vi "simArbSignal_rampUp.vi"(8 "error in (no error)":errorcluster, 9 "Reset":bool, 10 "Next Value":bool=TRUE) -> (0 "error out":errorcluster, 2 "Data Valid":bool, 3 "Signal":dynamicdata(graph)=[{"t0"=timestamp(0 s since 1904-01-01), "dt"=0.5, "Y"=array[3614 elements], "attributes"=variant("NI_ChannelName"=variant(string "Signal"))}])   [LabVIEW 2017]
doc: "Simulates a signal that you define.\n--------------------\n\nThis Express VI is configured as follows:\n\nMode: Packet (The whole waveform each run)\nCurve Specifications: Hold last value"
panel:
  in  "Repeat":bool
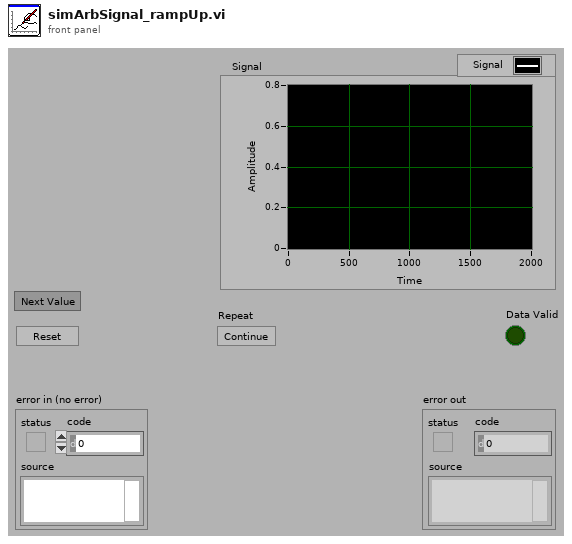
[diagram p1: front panel]
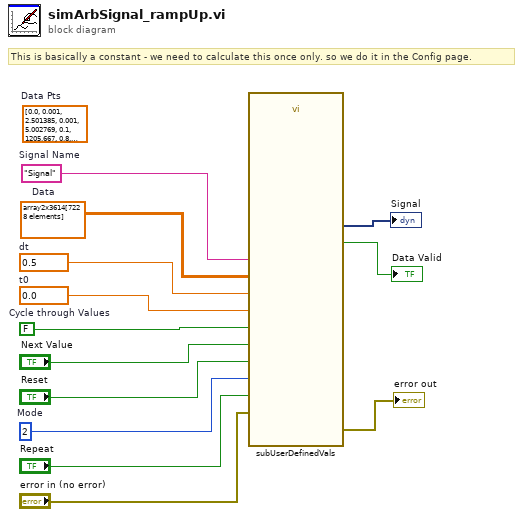
[diagram p0: block diagram]
diagram:
  (unwired) dbl[][] [[0.0, 0.001], [2.501385, 0.001], [5.002769, 0.1], [1205.667, 0.8], [1806.0, 0.0], [1806.5, 0.0]]  # Data Pts
  w4 = 2  # Mode
  w6 = FALSE  # Cycle through Values
  w11 = dbl[][] array2x3614[7228 elements]  # Data
  w7 = 0.0  # t0
  w8 = 0.5  # dt
  w13 = "Signal"  # Signal Name
  # "This is basically a constant - we need to calculate this once only. so we do it in the Config page."
  n1 = call <vilib>:"subUserDefinedVals.vi"("t0"=w7, "Next Value"="Next Value", "Mode"=w4, "dt"=w8, "error in (no error)"="error in (no error)", "Array"=w11, "Signal Name"=w13, "Cycle through Values"=w6, "Repeat"="Repeat", "Reset"="Reset") -> ("Signal"=→"Signal":dynamicdata, "error out"=→"error out":errorcluster, "Data Valid"=→"Data Valid":bool)  [unwired: 3 in]
